vi "Check Data.vi"(8 "error IO":errorcluster, 11 "LV Argument Parser in":refnum<class "LV Argument Parser.lvclass">) -> (0 "error out":errorcluster, 2 "Output":string, 3 "LV Argument Parser out":refnum<class "LV Argument Parser.lvclass">)   [LabVIEW 2020, in "LV ArgParse.lvlib" / "LV Argument Parser.lvclass"]
uses:
  LV Argument Parser.lvclass
  <vilib>/Utility/error.llb/Error Cluster From Error Code.vi
  <vilib>/ErrorRing/Error Ring.xnode
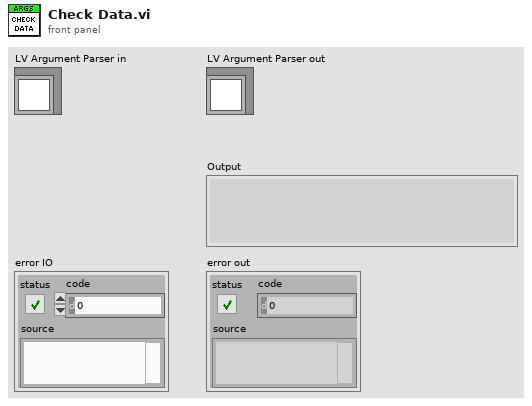
[diagram p1: front panel]
types:
  T1 = enum16{"unknown argument", "invalid argument type", "wrong argument count", "missing required argument"}
  T2 = typedef "LV ArgParse.lvlib/LV Argument Parser.lvclass/Argument Definition.ctl" = cluster{"Name":string, "short (positional)":string, "long (positional)":string, "action":enum16{"store", "store-const", "store-false", "store-true", "append", "append-const", "count", "help", "version"}, "choices":string[], "const":string, "default":string, "dest (=name)":string, "help":string, "Number":i32, "Required":bool, "Type":enum16{"String", "Int", "UInt", "Float", "Bool", "Date", "Path"}}
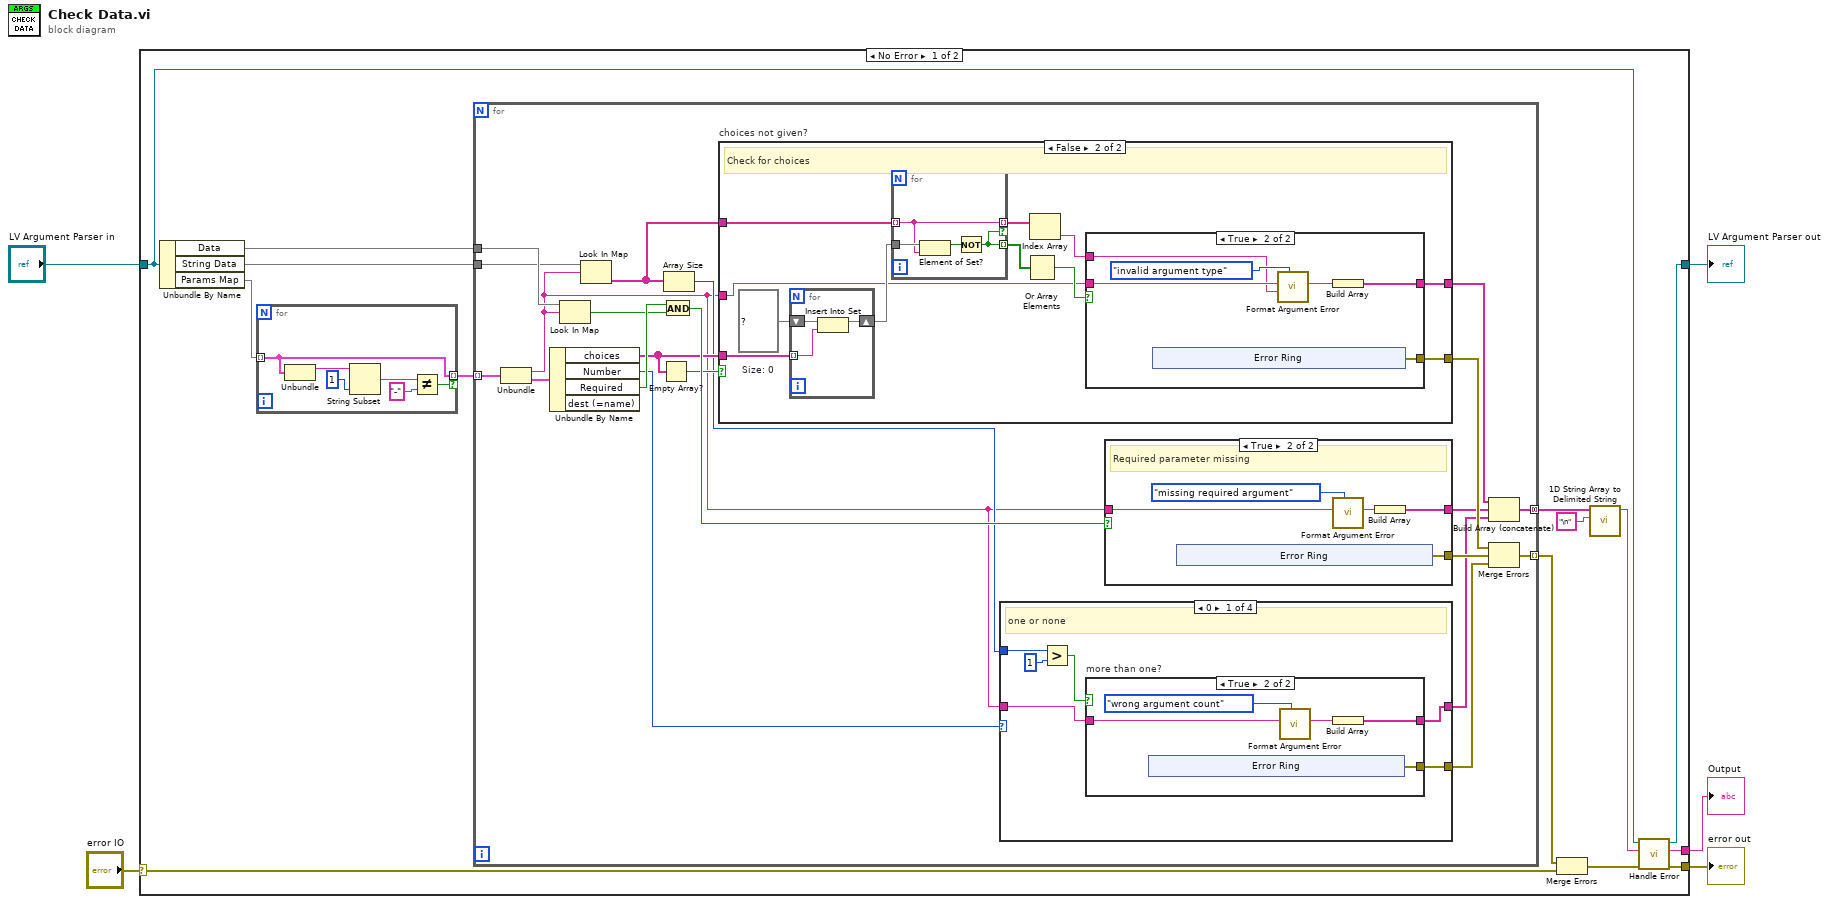
[diagram p0: block diagram]
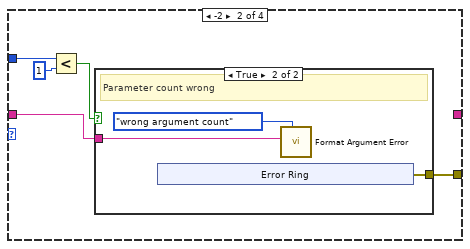
[diagram p3: hidden frame]
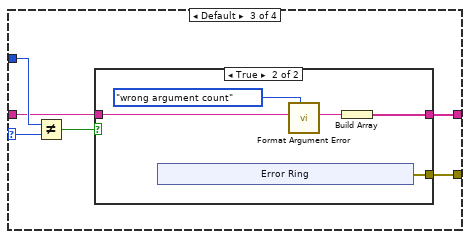
[diagram p5: hidden frame]
diagram:
  n1 = case shown="No Error" "error IO" {
    selector: "error IO" -> [w16 w127]
    tunnel: [w10 w127] -> w5
    tunnel: "LV Argument Parser in" -> [w12 w126]
    tunnel: [w11 w126] -> w2
    tunnel: [w8 _] -> w1
    frame No Error {
      n2 = Unbundle By Name(w12) -> ("Data"=w18:map{string, variant[]}, "String Data"=w17:map{string, string[]}, "Params Map"=w7:map{string, T2})
      n3 = for {
        tunnel: w7 -> [w21] mode=indexing
        tunnel: [w21] -> w6 mode=indexing if=w20
        n4 = Unbundle(w21) -> (w25:string)  [unwired: 1 out]
        n5 = String Subset(string=w25, length (rest)=1 ("length (rest)")) -> (substring=w23:string)  [unwired: 1 in]
        n6 = Not Equal?(x=w23, y="-") -> (x != y?=w20:bool)
      }
      n7 = for {
        tunnel: w18 -> [w44]
        tunnel: w6 -> [w46] mode=indexing
        tunnel: w17 -> [w43]
        tunnel: [w38] -> w19 mode=indexing
        tunnel: [w27] -> w15 mode=concatenating
        n8 = Unbundle(w46) -> (w26:string, "Argument Definition"=w45:T2)
        n9 = Unbundle By Name(w45) -> ("choices"=w33:string[], "Number"=w36:i32, "Required"=w41:bool)  [unwired: 1 out]
        n10 = Look In Map(map=w44, key=w26) -> (key not found?=w40:bool)  [unwired: 1 in, 1 out]
        n11 = Look In Map(map=w43, key=w26) -> (value=w32:string[])  [unwired: 1 in, 1 out]
        n12 = Empty Array?(array=w33) -> (empty?=w35:bool)
        n13 = And(x=w41, y=w40) -> (x .and. y?=w39:bool)
        n14 = Array Size(array=w32) -> (size(s)=w31:i32)
        n15 = case "choices not given?" shown="False" w35 {
          tunnel: w32 -> [_ w108]
          tunnel: w33 -> [_ w107]
          tunnel: [_ w103] -> w42
          tunnel: w26 -> [_ w101]
          tunnel: [_ w100] -> w30
          frame True {
          }
          frame False {
            w106 = set{string} {}  # Size: 0
            # "Check for choices"
            n16 = for {
              tunnel: w107 -> [w120] mode=indexing
              shift-right: [w119] -> w105
              shift-left: w106 -> [w121]
              n17 = Insert Into Set(10:w120, 11:w121) -> (3:w119:set{string})  [unwired: 1 out]
            }
            n18 = for {
              tunnel: w108 -> [w123] mode=indexing
              tunnel: w105 -> [w125]
              tunnel: [w122] -> w104 mode=indexing
              tunnel: [w123] -> w99 mode=indexing if=w122
              n19 = Element of Set?(10:w123, 11:w125) -> (3:w124:bool)
              n20 = Not(x=w124) -> (.not. x?=w122:bool)
            }
            n21 = Or Array Elements(Boolean array=w104) -> (logical OR=w102:bool)
            n22 = Index Array(array=w99) -> (element=w98:string)  [unwired: 1 in]
            n23 = case shown="True" w102 {
              tunnel: [_ w114] -> w103
              tunnel: w101 -> [_ w113]
              tunnel: [_ w110] -> w100
              tunnel: w98 -> [_ w109]
              frame False {
              }
              frame True {
                n24 = xnode "Error Ring"() -> ("error out"=w114:errorcluster)
                n25 = call "Format Argument Error.vi"("Error Type"=T1."invalid argument type", "Value"=w109, "Name"=w113) -> ("String"=w111:string)  [unwired: 8 in]
                n26 = Build Array(w111) -> (w110:string[])
              }
            }
          }
        }
        n27 = case shown="0" w36 {
          selector: w36 -> [_ _ w78 _]
          tunnel: w31 -> [w52 w66 w79 _]
          tunnel: [w49 w63 w76 _] -> w34
          tunnel: w26 -> [w48 w62 w75 _]
          tunnel: [w47 _ w74 _] -> w28
          frame 0 {
            # "one or none"
            n28 = Greater?(x=w52, y=1) -> (0:w50:bool)
            n29 = case "more than one?" shown="True" w50 {
              tunnel: [_ w57] -> w49
              tunnel: w48 -> [_ w56]
              tunnel: [_ w54] -> w47
              frame False {
              }
              frame True {
                n30 = xnode "Error Ring"() -> ("error out"=w57:errorcluster)
                n31 = call "Format Argument Error.vi"("Error Type"=T1."wrong argument count", "Name"=w56) -> ("String"=w55:string)  [unwired: 9 in]
                n32 = Build Array(w55) -> (w54:string[])
              }
            }
          }
          frame -2 {
            n33 = Less?(x=w66, y=1) -> (x < y?=w64:bool)
            n34 = case shown="True" w64 {
              tunnel: [_ w69] -> w63
              tunnel: w62 -> [_ w68]
              frame False {
              }
              frame True {
                # "Parameter count wrong"
                n35 = xnode "Error Ring"() -> ("error out"=w69:errorcluster)
                n36 = call "Format Argument Error.vi"("Error Type"=T1."wrong argument count", "Name"=w68) -> ()  [unwired: 9 in, 1 out]
              }
            }
          }
          frame Default {
            n37 = Not Equal?(x=w79, y=w78) -> (x != y?=w77:bool)
            n38 = case shown="True" w77 {
              tunnel: [_ w84] -> w76
              tunnel: w75 -> [_ w83]
              tunnel: [_ w80] -> w74
              frame False {
              }
              frame True {
                n39 = xnode "Error Ring"() -> ("error out"=w84:errorcluster)
                n40 = call "Format Argument Error.vi"("Error Type"=T1."wrong argument count", "Name"=w83) -> ("String"=w81:string)  [unwired: 9 in]
                n41 = Build Array(w81) -> (w80:string[])
              }
            }
          }
          frame -1 {
            # "any number"
          }
        }
        n42 = case shown="True" w39 {
          tunnel: [_ w93] -> w37
          tunnel: w26 -> [_ w92]
          tunnel: [_ w89] -> w29
          frame False {
          }
          frame True {
            # "Required parameter missing"
            n43 = xnode "Error Ring"() -> ("error out"=w93:errorcluster)
            n44 = call "Format Argument Error.vi"("Error Type"=T1."missing required argument", "Name"=w92) -> ("String"=w90:string)  [unwired: 9 in]
            n45 = Build Array(w90) -> (w89:string[])
          }
        }
        n46 = Build Array (concatenate)(w30, w29, w28) -> (w27:string[])
        n47 = Merge Errors(w42, w37, w34) -> (w38:errorcluster)
      }
      n48 = Merge Errors(w19, w16) -> (w9:errorcluster)
      n49 = call <vilib>:"1D String Array to Delimited String.vi"("delimiter"="\n", "string array"=w15) -> ("delimited string"=w13:string)  [unwired: 9 in]
      n50 = call "Handle Error.vi"("error in (no error)"=w9, "delimited string"=w13, "LV Argument Parser in"=w12) -> ("error out"=w10:errorcluster, "Output"=w8:string, "LV Argument Parser out"=w11:refnum<class "LV Argument Parser.lvclass">)  [unwired: 6 in]
    }
    frame Error {
    }
  }
  "error out" <- w5
  "LV Argument Parser out" <- w2
  "Output" <- w1
